vi "Array Test.vi"(8 "error in (no error)":errorcluster) -> (0 "error out":errorcluster, 2 "Pass?":bool, 3 "Test VIs Run":refnum<vi>[](array[refnum]))   [LabVIEW 2020]
doc: "This VI template can be used for executing testing VIs found in the same directory as this VI with names of the form <this VI's name> - *.vi. Note that this VI does not close the references for the VIs called, but passed them out for use in determining which VIs have been tested.\n\nCoded by Douglas A. Femec, January 24, 2006.\n\nCopyright (c) 2005-2006 MKS Instruments, Inc.\nAll rights reserved."
uses:
  Test VI Refnum.ctl
panel:
  in  "Generic VI Refnum":refnum<vi>
  in  "Test VI Refnum":T1
  # "Copyright (c) 2005-2006 MKS Instruments, Inc.\nAll rights reserved."
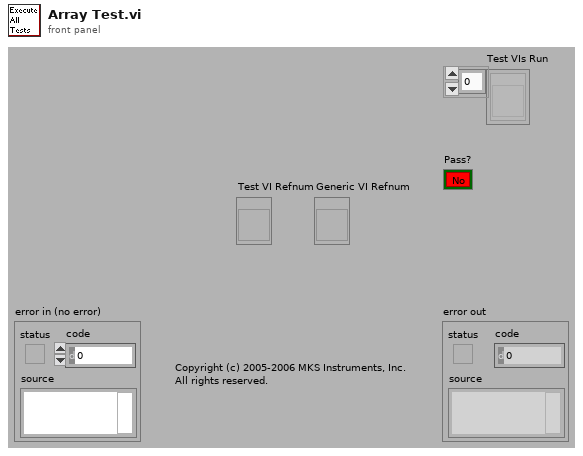
[diagram p1: front panel]
types:
  T1 = typedef "Test VI Refnum.ctl" = refnum<vi>
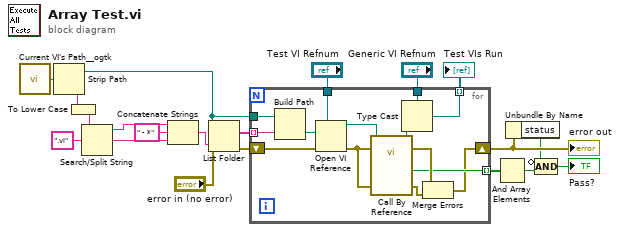
[diagram p0: block diagram]
diagram:
  n1 = call <userlib>:"Current VI's Path__ogtk.vi"() -> ("Current VI's Path (+ Relative)"=w20:path)  [unwired: 1 in]
  n2 = Strip Path(path=w20) -> (stripped path=w11:path, name=w19:string)
  n3 = To Lower Case(string=w19) -> (all lower case string=w17:string)
  n4 = Search/Split String(string=w17, search string/char (-)=".vi") -> (substring before match=w16:string, match + rest of string=w15:string)  [unwired: 1 in, 1 out]
  n5 = Concatenate Strings(w16, " - *" ("string"), w15) -> (w13:string)
  n6 = List Folder(path=w11, pattern=w13, error in="error in (no error)") -> (filenames=w12:string[], error out=w10:errorcluster)  [unwired: 1 in, 2 out]
  n7 = for {
    tunnel: w12 -> [w34] mode=indexing
    tunnel: w11 -> [w33]
    shift-right: [w24] -> w4
    shift-left: w10 -> [w29]
    tunnel: "Test VI Refnum" -> [w30]
    tunnel: [w26] -> w7 mode=indexing
    tunnel: [w22] -> w2 mode=indexing
    tunnel: "Generic VI Refnum" -> [w21]
    n8 = Build Path(base path=w33, name or relative path=w34) -> (appended path=w25:path)
    n9 = Open VI Reference(type specifier VI Refnum (for type only)=w30, vi path=w25, error in (no error)=w29) -> (vi reference=w32:T1, error out=w28:errorcluster)  [unwired: 3 in]
    n10 = call-by-ref "?"(reference=w32, error in=w28, "error in (no error)"=w28) -> (reference out=w23:T1, error out=w31:errorcluster, 0:"error out"=w27:errorcluster, "Pass?"=w26:bool)  [unwired: 9 in]
    n11 = Type Cast(type=w21, x=w23) -> (*(type *) &x=w22:refnum<vi>)
    n12 = Merge Errors(w31, w27) -> (w24:errorcluster)
  }
  "error out" <- w4
  "Test VIs Run" <- w2
  n13 = And Array Elements(Boolean array=w7) -> (logical AND=w6:bool)
  n14 = Unbundle By Name(w4) -> ("status"=w3:bool)
  n15 = Compound Arithmetic op=AND(invert w3, w6) -> (→"Pass?":bool)
